vi "写D+32位.vi"(8 "error out":errorcluster, 9 "输入数值":i32, 10 "输入地址D":i32, 11 "VISA resource name out":refnum<visa-resource-name>) -> (0 "error out 2":errorcluster caption="error out", 1 "连接的字符串":string, 2 "读取缓冲区":string, 3 "VISA resource name out 2":refnum<visa-resource-name>)   [LabVIEW 2018]
uses:
  <vilib>/Instr/_visa.llb/VISA Configure Serial Port (Instr).vi
panel:
  out "通讯延时":u32
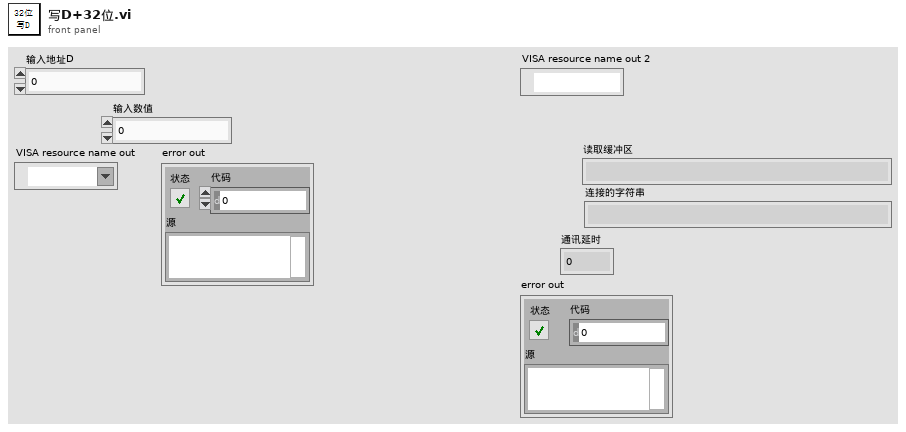
[diagram p1: front panel]
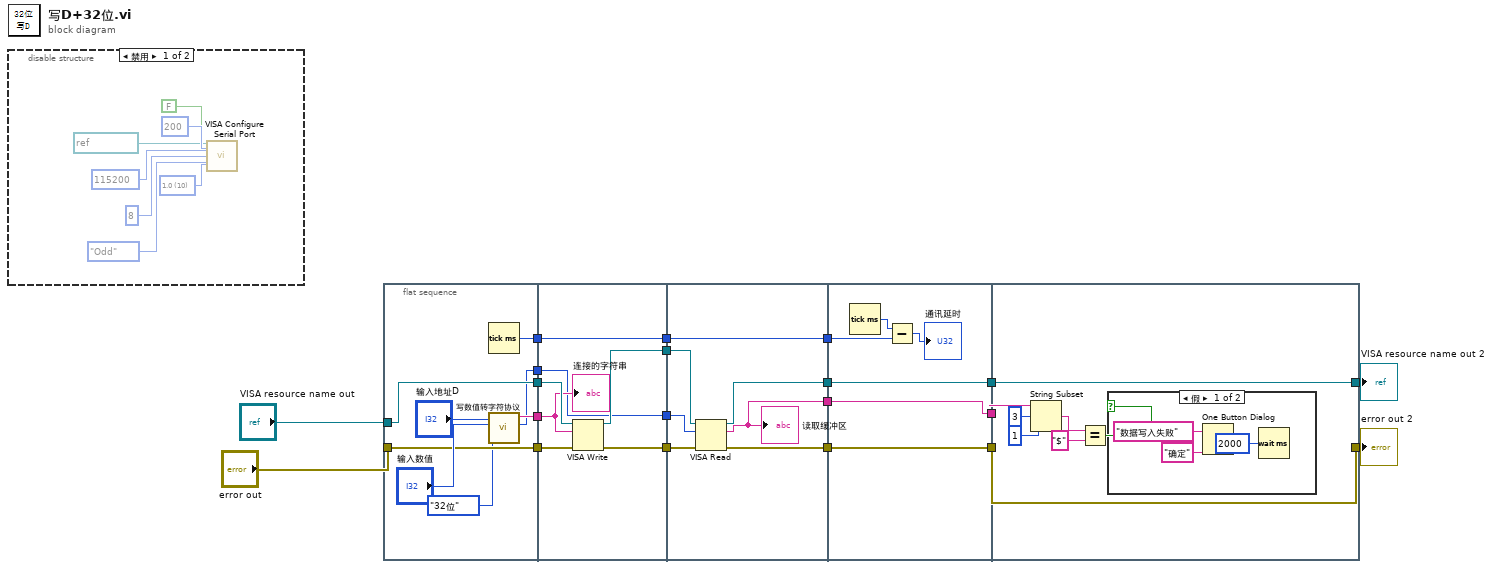
[diagram p0: block diagram]
diagram:
  n1 = disable-structure shown="禁用" {
    frame Disabled {
      w25 = u16 10 items=["1.0"=10, "1.5"=15, "2.0"=20] ("stop bits (10: 1 bit)")
      n2 = call-poly "VISA Configure Serial Port"("VISA resource name"=refnum<visa-resource-name> "COM3", "timeout (10sec)"=u32 200, "Enable Termination\nChar (T)"=FALSE ("Enable Termination\nChar (T)"), "baud rate (9600)"=u32 115200, "data bits (8)"=u16 8, "parity (0:none)"=enum16{"None", "Odd", "Even", "Mark", "Space"}."Odd", "stop bits (10: 1 bit)"=w25) -> ()  [unwired: 7 in, 2 out]
    }
    frame Enabled {
    }
  }
  n3 = flat-sequence {
    tunnel: "VISA resource name out" -> [w34]
    tunnel: "error out" -> [w33]
    tunnel: [w34] -> w20
    tunnel: [w33] -> w19
    tunnel: [w32] -> w18
    tunnel: [w31] -> w14
    tunnel: [w30] -> w13
    tunnel: w20 -> [w41]
    tunnel: w19 -> [w42]
    tunnel: w18 -> [w40]
    tunnel: [w39] -> w17
    tunnel: [w38] -> w16
    tunnel: [w37] -> w15
    tunnel: w14 -> [w37]
    tunnel: w13 -> [w36]
    tunnel: [w36] -> w12
    tunnel: w17 -> [w47]
    tunnel: w16 -> [w46]
    tunnel: w15 -> [w45]
    tunnel: w12 -> [w44]
    tunnel: [w49] -> w11
    tunnel: [w48] -> w10
    tunnel: [w44] -> w9
    tunnel: [w43] -> w5
    tunnel: w11 -> [w55]
    tunnel: w10 -> [w54]
    tunnel: w9 -> [w52]
    tunnel: [w55] -> w8
    tunnel: [w54] -> w7
    tunnel: [w50] -> w6
    tunnel: w5 -> [w50]
    tunnel: [w62] -> w1
    tunnel: [w63] -> w2
    tunnel: w8 -> [w63]
    tunnel: w7 -> [w62]
    tunnel: w6 -> [w61]
    frame #0 {
      n4 = Tick Count (ms)() -> (millisecond timer value=w30:u32)
      n5 = call "写数值转字符协议.vi"("枚举"=enum16{"16位", "32位"}."32位", "输入数值"="输入数值", "输入地址"="输入地址D") -> ("返回字节数"=w31:u16, "连接的字符串"=w32:string)  [unwired: 7 in]
    }
    frame #1 {
      n6 = VISA Write(VISA resource name=w41, write buffer=w40, error in (no error)=w42) -> (VISA resource name out=w39:refnum<visa-resource-name>, error out=w38:errorcluster)  [unwired: 1 out]
      "连接的字符串" <- w40
    }
    frame #2 {
      n7 = VISA Read(VISA resource name=w47, byte count=w45, error in (no error)=w46) -> (VISA resource name out=w49:refnum<visa-resource-name>, read buffer=w43:string, error out=w48:errorcluster)  [unwired: 1 out]
      "读取缓冲区" <- w43
    }
    frame #3 {
      n8 = Tick Count (ms)() -> (millisecond timer value=w53:u32)
      n9 = Subtract(x=w53, y=w52) -> (x-y=→"通讯延时":u32)
    }
    frame #4 {
      n10 = String Subset(string=w61, offset (0)=3 ("偏移量(0)"), length (rest)=1 ("长度（剩余）")) -> (substring=w58:string)
      n11 = Equal?(x=w58, y="$") -> (x = y?=w56:bool)
      n12 = case shown="假" w56 {
        frame False {
          n13 = One Button Dialog(message="数据写入失败" ("消息"), button name ("OK")="确定" ("按钮名称（“确定”）")) -> ()  [unwired: 1 out]
          n14 = Wait (ms)(milliseconds to wait=u32 2000 ("等待时间（毫秒）")) -> ()  [unwired: 1 out]
        }
        frame True {
        }
      }
    }
  }
  "VISA resource name out 2" <- w2
  "error out 2" <- w1
